vi "Operator.vi"(8 "Aquiring?":bool, 9 "Photoeye":bool, 11 "JoystickDevRef in":T2) -> (1 "Output":T1, 3 "JoystickDevRef out":T2)   [LabVIEW 2015]
uses:
  <vilib>/Rock Robotics/WPI/Joystick/WPI_JoystickDevRef.ctl
  <vilib>/Rock Robotics/WPI/Joystick/WPI_JoystickDeviceEnum.ctl
  <vilib>/Rock Robotics/Network Tables/NT Write Numeric Array.vi
  <vilib>/Rock Robotics/Network Tables/NT Write Boolean Array.vi
  <vilib>/ptbypt/NI_PtbyPt.lvlib
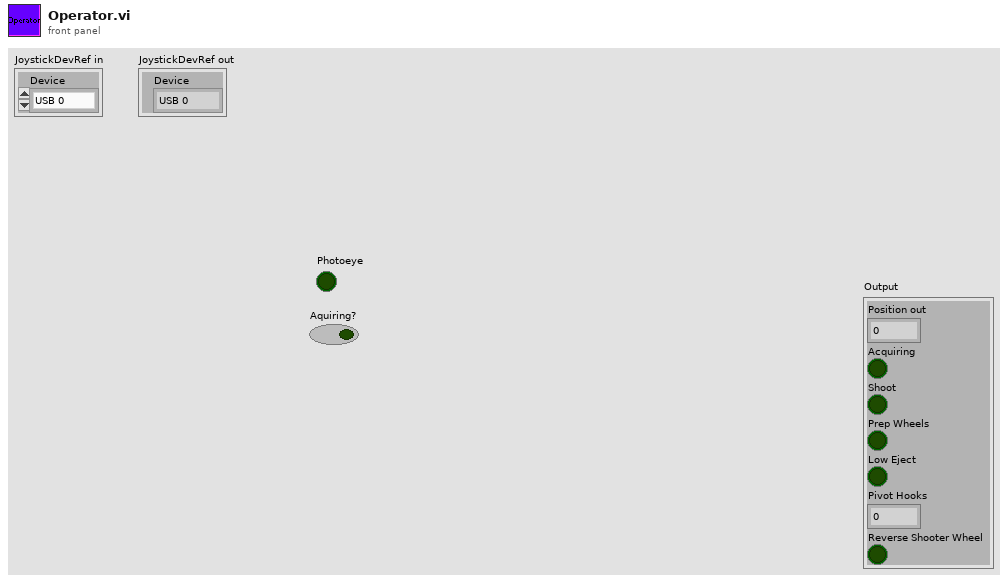
[diagram p1: front panel]
types:
  T1 = cluster{"Position out":dbl, "Acquiring":bool, "Shoot":bool, "Prep Wheels":bool, "Low Eject":bool, "Pivot Hooks":dbl, "Reverse Shooter Wheel":bool}
  T2 = typedef "WPI_JoystickDevRef.ctl" = cluster{"Device":T3}
  T3 = typedef "WPI_JoystickDeviceEnum.ctl" = enum16{"USB 0", "USB 1", "USB 2", "USB 3", "USB 4", "USB 5"}
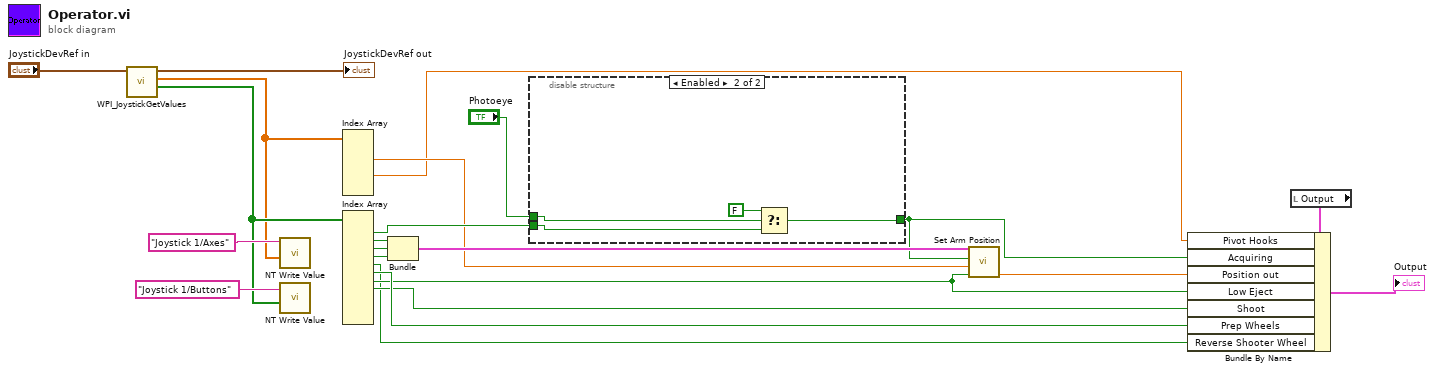
[diagram p0: block diagram]
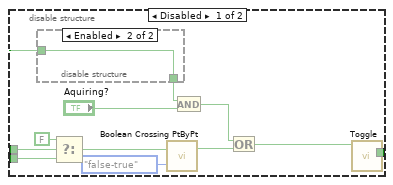
[diagram p2: hidden frame]
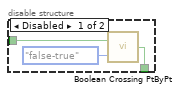
[diagram p3: hidden frame]
diagram:
  n1 = call <vilib>:"WPI_JoystickGetValues.vi"("JoystickDevRef"="JoystickDevRef in") -> ("Buttons"=w20:bool[], "Axes"=w19:dbl[], "JoystickDevRef"=→"JoystickDevRef out":T2)  [unwired: 6 in, 2 out]
  n2 = call-poly <vilib>:"NT Write Value.vi"("Numeric Array"=w19, "Name"="Joystick 1/Axes") -> ()  [unwired: 9 in, 1 out]
  n3 = call-poly <vilib>:"NT Write Value.vi"("Boolean Array"=w20, "Name"="Joystick 1/Buttons") -> ()  [unwired: 9 in, 1 out]
  n4 = Index Array(array=w19) -> (element #2=w2:dbl, element #4=w1:dbl)  [unwired: 6 in, 4 out]
  n5 = Index Array(array=w20) -> (element #1=w4:bool, element #2=w16:bool, element #3=w15:bool, element #4=w14:bool, element #5=w3:bool, element #6=w9:bool, element #7=w7:bool, element #8=w8:bool)  [unwired: 12 in, 4 out]
  n6 = Bundle(w16, w15, w14) -> (w13:cluster{bool, bool, bool})  [unwired: 1 in]
  n7 = disable-structure shown="Enabled" {
    disable-tunnel: [w31 w41] -> w6
    disable-tunnel: "Photoeye" -> [w28 w39]
    disable-tunnel: w4 -> [w27 w40]
    frame Disabled {
      n8 = disable-structure shown="Enabled" {
        disable-tunnel: [w35 w37] -> w33
        disable-tunnel: w28 -> [w34 w37]
        frame Disabled {
          n9 = call <vilib>:"Boolean Crossing PtByPt.vi"("direction"=enum16{"either", "false-true", "true-false"}."false-true", "input"=w34) -> ("crossing"=w35:bool)  [unwired: 1 in]
        }
        frame Enabled {
        }
      }
      n10 = Select(t=FALSE, s=w28, f=w27) -> (s? t:f=w24:bool)
      n11 = call <vilib>:"Boolean Crossing PtByPt.vi"("direction"=enum16{"either", "false-true", "true-false"}."false-true", "input"=w24) -> ("crossing"=w23:bool)  [unwired: 1 in]
      n12 = And(x=w33, y="Aquiring?") -> (x .and. y?=w30:bool)
      n13 = Or(x=w30, y=w23) -> (x .or. y?=w29:bool)
      n14 = call "Toggle.vi"("Input"=w29) -> ("output"=w31:bool)  [unwired: 10 in]
    }
    frame Enabled {
      n15 = Select(t=FALSE, s=w39, f=w40) -> (s? t:f=w41:bool)
    }
  }
  n16 = call "Set Arm Position.vi"("Button  States"=w13, "Acquiring"=w6, "Right Stick Value"=w2, "Low Eject"=w7) -> ("Position out"=w10:dbl)  [unwired: 6 in]
  n17 = local read "Output"() -> (w11:T1)
  n18 = Bundle By Name(cluster=w11, "Pivot Hooks"=w1, "Acquiring"=w6, "Position out"=w10, "Low Eject"=w7, "Shoot"=w8, "Prep Wheels"=w9, "Reverse Shooter Wheel"=w3) -> (→"Output":T1)
